vi "to string.vi"(8 "error in":errorcluster, 11 "fixed channel configuration in":refnum<class "AppStateMachine configuration.lvclass">) -> (0 "error out":errorcluster, 1 "data":string, 2 "version":string, 3 "fixed channel configuration out":refnum<class "AppStateMachine configuration.lvclass">)   [LabVIEW 2017, in "AppStateMachine configuration.lvclass"]
doc: "Provides an interface for saving a module configuration to a file or other serialized data source. It is recommended that all children of this class store data in two sets--data required for its own initialization, and any data required for parent initialization--and that each implementation uses the <b>Call Parent Method</b> primitive to serialize parent information.\nNI Tag Bus Module Framework 1.0.3.43\nNI Systems Engineering"
uses:
  AppStateMachine configuration.lvclass
  AppStateMachine configuration.lvclass/AppStateMachine configuration.ctl
  <vilib>/NI/JSON Support for LabVIEW/JSON Data Classes/JSON Object/New JSON Object (Empty).vi
  <vilib>/NI/JSON Support for LabVIEW/JSON Data Classes/JSON Object/Insert Key Value Pair (Single Numeric).vi
  <vilib>/NI/DCAF/Tag Editor Core/control module/configuration/control module configuration.lvclass
  <vilib>/NI/JSON Support for LabVIEW/JSON Data Classes/JSON Object/JSON Object.lvclass
  <vilib>/NI/Configuration Framework/serializable configuration/NISE_CEF_serializable configuration.lvclass
  <vilib>/NI/JSON Support for LabVIEW/JSON Data Classes/JSON Helper/JSON Helper.lvclass
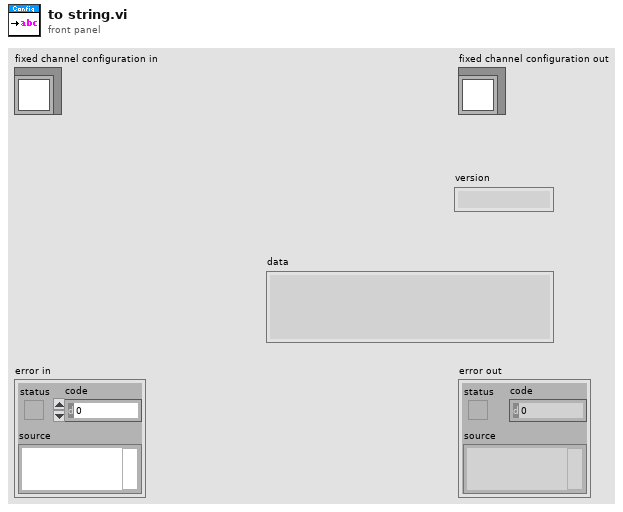
[diagram p1: front panel]
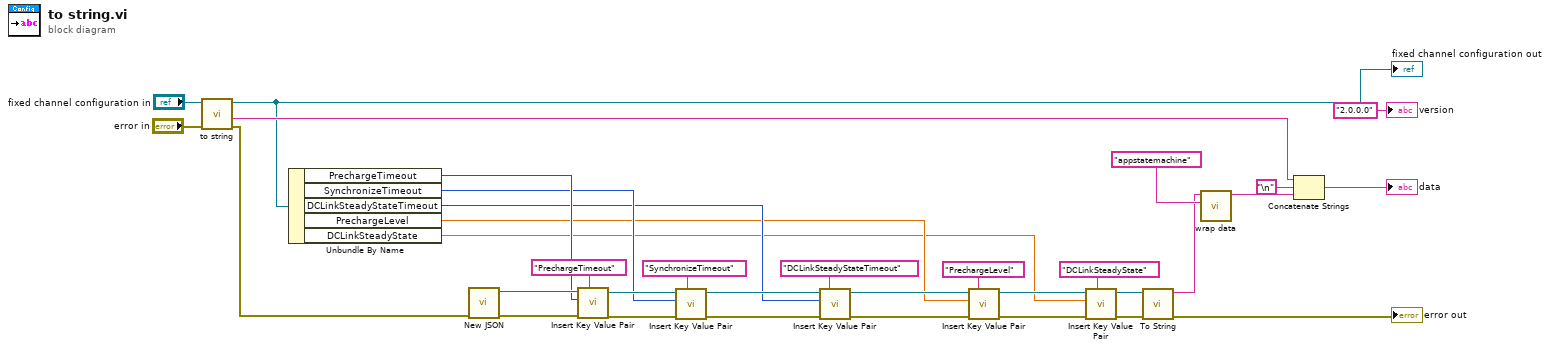
[diagram p0: block diagram]
diagram:
  n1 = call-parent "to string.vi"("error in"="error in", "fixed channel configuration in"="fixed channel configuration in") -> ("error out"=w6:errorcluster, "data"=w30:string, "fixed channel configuration out"=w27:refnum<class "AppStateMachine configuration.lvclass">)  [unwired: 6 in, 1 out]
  "fixed channel configuration out" <- w27
  n2 = Unbundle By Name(w27) -> ("PrechargeTimeout"=w24:u32, "SynchronizeTimeout"=w20:u32, "DCLinkSteadyStateTimeout"=w16:u32, "PrechargeLevel"=w11:dbl, "DCLinkSteadyState"=w7:dbl)
  n3 = call-poly <vilib>:"New JSON.vi"("error in (no error)"=w6) -> ("error out"=w26:errorcluster, "JSON Object out"=w25:refnum<class "JSON Object.lvclass">)  [unwired: 9 in]
  n4 = call-poly <vilib>:"Insert Key Value Pair.vi"("key"="PrechargeTimeout", "error in (no error)"=w26, "value"=w24, "JSON Object in"=w25) -> ("error out"=w21:errorcluster, "JSON Object out"=w22:refnum<class "JSON Object.lvclass">)  [unwired: 5 in, 1 out]
  n5 = call-poly <vilib>:"Insert Key Value Pair.vi"("key"="SynchronizeTimeout", "error in (no error)"=w21, "value"=w20, "JSON Object in"=w22) -> ("error out"=w15:errorcluster, "JSON Object out"=w18:refnum<class "JSON Object.lvclass">)  [unwired: 5 in, 1 out]
  n6 = call-poly <vilib>:"Insert Key Value Pair.vi"("key"="DCLinkSteadyStateTimeout", "error in (no error)"=w15, "value"=w16, "JSON Object in"=w18) -> ("error out"=w13:errorcluster, "JSON Object out"=w14:refnum<class "JSON Object.lvclass">)  [unwired: 5 in, 1 out]
  n7 = call-poly <vilib>:"Insert Key Value Pair.vi"("key"="PrechargeLevel", "error in (no error)"=w13, "value"=w11, "JSON Object in"=w14) -> ("error out"=w8:errorcluster, "JSON Object out"=w9:refnum<class "JSON Object.lvclass">)  [unwired: 5 in, 1 out]
  n8 = call-poly <vilib>:"Insert Key Value Pair.vi"("key"="DCLinkSteadyState", "error in (no error)"=w8, "value"=w7, "JSON Object in"=w9) -> ("error out"=w4:errorcluster, "JSON Object out"=w5:refnum<class "JSON Object.lvclass">)  [unwired: 5 in, 1 out]
  n9 = call-dynamic "To String.vi"("error in (no error)"=w4, "JSON Object in"=w5) -> ("error out"=→"error out":errorcluster, "String"=w3:string)  [unwired: 8 in]
  n10 = call <vilib>:"wrap data.vi"("identifier"="appstatemachine", "data to wrap"=w3) -> ("wrapped data"=w31:string)  [unwired: 9 in]
  n11 = Concatenate Strings(w30, "\n", w31) -> (→"data":string)
  "version" <- "2.0.0.0" ("version")
